vi "ctldatasend.vi"(11 "Data":dbl[](array[numeric])) -> ()   [LabVIEW 2015]
uses:
  multi_queue_enum.ctl
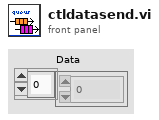
[diagram p1: front panel]
types:
  T1 = typedef "multi_queue_enum.ctl" = enum16{"Noop", "add queues", "Send Pro1", "Send data", "Get Pro1", "Get data", "Flush Pro1", "Flush data", "Destroy Pro1", "Destroy data"}
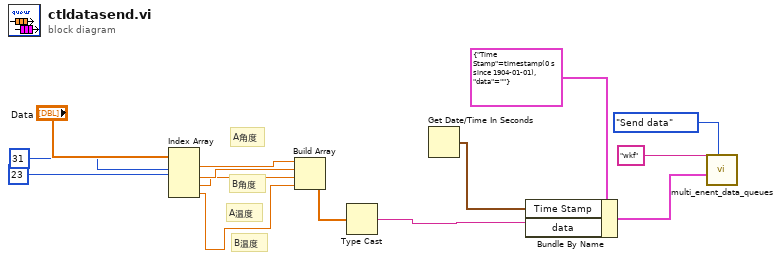
[diagram p0: block diagram]
diagram:
  # "B温度"
  # "A温度"
  # "B角度"
  # "A角度"
  n1 = Index Array(array="Data", index #1=31 ("index"), index #2=23 ("index")) -> (element #1=w6:dbl, element #2=w5:dbl, element #3=w4:dbl, element #4=w3:dbl)  [unwired: 2 in]
  n2 = Build Array(w6, w5, w4, w3) -> (w2:dbl[])
  n3 = Type Cast(x=w2) -> (*(type *) &x=w1:string)  [unwired: 1 in]
  n4 = Get Date/Time In Seconds() -> (seconds since 1Jan1904=w10:timestamp)
  n5 = Bundle By Name(cluster=cluster{"Time Stamp":timestamp, "data":string} {"Time Stamp"=timestamp(0 s since 1904-01-01), "data"=""} ("data"), "Time Stamp"=w10, "data"=w1) -> (w9:cluster{"Time Stamp":timestamp, "data":string})
  n6 = call "multi_enent_data_queues.vi"("Mode"=multi_queue_enum."Send data", "data"=w9, "name"="wkf") -> ()  [unwired: 4 in, 5 out]
